vi "String to GU Number Array.vi"(1 "GU Numbers String":string) -> (0 "GU Numbers Array":i32[](array[numeric]))   [LabVIEW 2020, in "GUCalibration2.lvlib"]
uses:
  GUCalibration2.lvlib
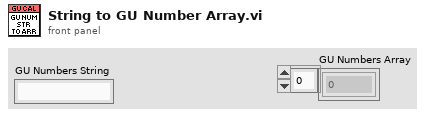
[diagram p1: front panel]
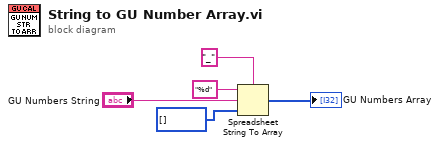
[diagram p0: block diagram]
diagram:
  n1 = Spreadsheet String To Array(delimiter (Tab)="_", format string="%d", spreadsheet string="GU Numbers String", array type (2D Dbl)=i32[] []) -> (array=→"GU Numbers Array":i32[])
